vi "Ev Num.vi"(8 "error in (no error)":errorcluster, 11 "Pic Json Generator in":refnum<class "Pic Json Generator.lvclass">) -> (0 "error out":errorcluster, 3 "Pic Json Generator out":refnum<class "Pic Json Generator.lvclass">)   [LabVIEW 2018, in "Pic Json Generator.lvlib" / "Pic Json Generator.lvclass"]
uses:
  Pic Json Generator.lvclass
  Pic Json Generator.lvclass/Pic Json Generator.ctl
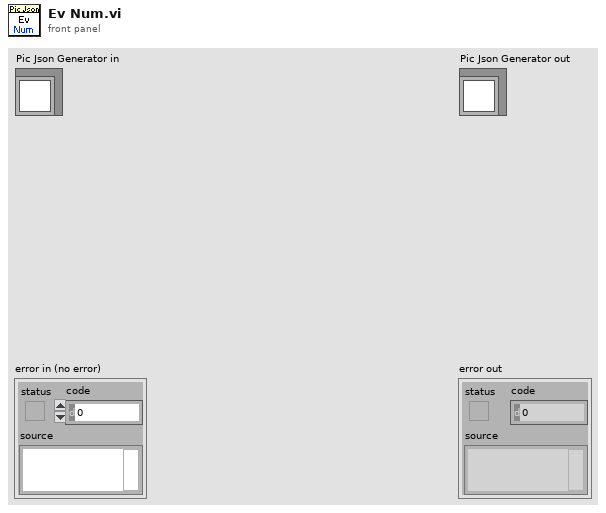
[diagram p1: front panel]
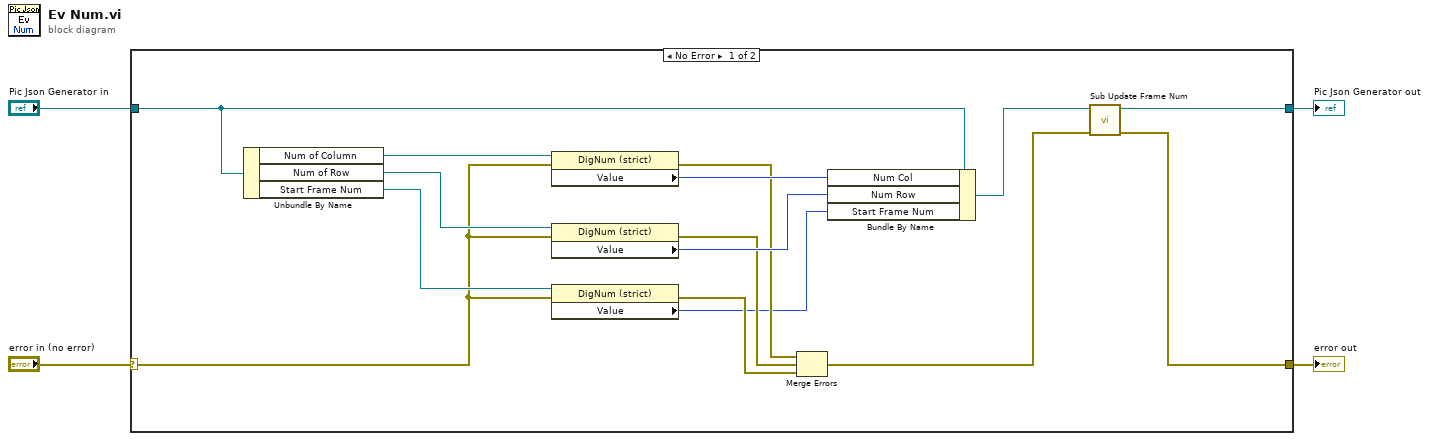
[diagram p0: block diagram]
diagram:
  n1 = case shown="No Error" "error in (no error)" {
    selector: "error in (no error)" -> [w11 w21]
    tunnel: [w5 w21] -> w3
    tunnel: [w7 w20] -> w1
    tunnel: "Pic Json Generator in" -> [w19 w20]
    frame No Error {
      n2 = Unbundle By Name(w19) -> ("Num of Column"=w18:refnum<vi>, "Num of Row"=w17:refnum<vi>, "Start Frame Num"=w12:refnum<vi>)
      n3 = property class="DigNum (strict)"(reference=w18, error in=w11) -> (error out=w14:errorcluster, "Value"=w16:u32)  [unwired: 1 out]
      n4 = property class="DigNum (strict)"(reference=w17, error in=w11) -> (error out=w13:errorcluster, "Value"=w15:u32)  [unwired: 1 out]
      n5 = property class="DigNum (strict)"(reference=w12, error in=w11) -> (error out=w10:errorcluster, "Value"=w9:u32)  [unwired: 1 out]
      n6 = Merge Errors(w14, w13, w10) -> (w6:errorcluster)
      n7 = Bundle By Name(cluster=w19, "Num Col"=w16, "Num Row"=w15, "Start Frame Num"=w9) -> (w8:refnum<class "Pic Json Generator.lvclass">)
      n8 = call "Sub Update Frame Num.vi"("error in (no error)"=w6, "Pic Json Generator in"=w8) -> ("error out"=w5:errorcluster, "Pic Json Generator out"=w7:refnum<class "Pic Json Generator.lvclass">)  [unwired: 8 in]
    }
    frame Error {
    }
  }
  "error out" <- w3
  "Pic Json Generator out" <- w1
